vi "StorageXMutationAddTermForClose.vi"(1 "Node type":T4(ring), 2 "TermSpecs in":T1[](array[typedef])) -> (0 "TermSpecs out":T1[](array[typedef]))   [LabVIEW 2017]
uses:
  <vilib>/Platform/storage/lvStorage.llb/TerminalDef.ctl
  <vilib>/Platform/storage/lvStorage.llb/_TerminalStyle.ctl
  <vilib>/Utility/XNodeSupport.llb/XRect32.ctl
  <vilib>/Platform/storage/lvStorage.llb/_dataTypeEnumForTerminals.ctl
panel:
  in  "Name":string="file path"
  in  "terminalDef":T1={"direction"=enum."Input", "typeDescriptor"="", "color"=0, "oldTerm"=0, "style"=enum."Express", "optional"=FALSE, "bounds"={"t"=0, "l"=0, "b"=138, "r"=96}, "termRefs"=[], "Name"="", "Data"=variant, "wiredTypeDescriptor"=""}
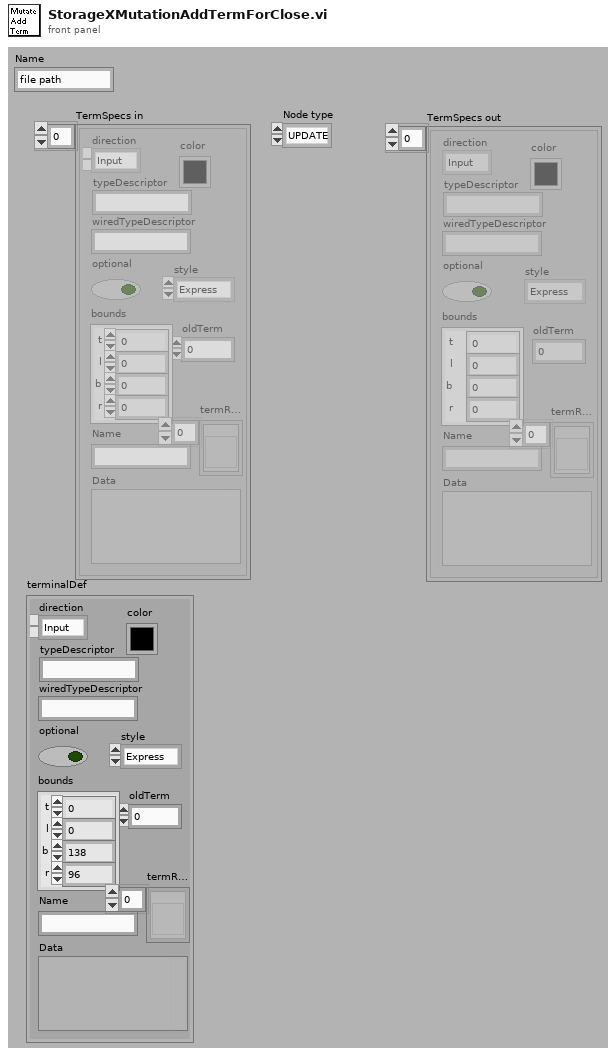
[diagram p1: front panel]
types:
  T1 = typedef "TerminalDef.ctl" = cluster{"direction":enum16{"Input", "Output"}, "typeDescriptor":string, "color":u32, "oldTerm":i32, "style":T2, "optional":bool, "bounds":T3, "termRefs":refnum<vi>[], "Name":string, "Data":variant, "wiredTypeDescriptor":string}
  T2 = typedef "_TerminalStyle.ctl" = enum16{"Express", "Collapsed", "Internal"}
  T3 = typedef "XRect32.ctl" = cluster{"t":i32, "l":i32, "b":i32, "r":i32}
  T4 = enum16{"UPDATE", "READ", "QUERY", "CREATE CHILD", "CREATE", "CONNECT", "DISCONNECT"}
  T5 = typedef "_dataTypeEnumForTerminals.ctl" = enum16{"Data Storage", "Data Object", "Root", "Channel", "Error in", "Error out", "Storage Location (path)", "Storage Location (string)", "Storage Format", "Overwrite options (enum)", "Append / Replace (enum)", "index", "count", "Comparison (enum)", "Signal", "Channelgroup", "Cluster", "DBL", "SGL", "I32", "I16", "U8", "TIME", "STRING", "ENUM", "waveform", "DDT", "DAQmx Channel"}
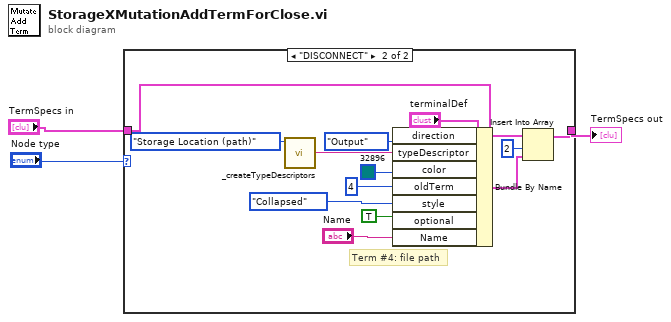
[diagram p0: block diagram]
diagram:
  n1 = case shown="\"DISCONNECT\"" "Node type" {
    tunnel: "TermSpecs in" -> [w4 w8]
    tunnel: [w4 w5] -> w2
    frame Default {
    }
    frame "DISCONNECT" {
      # "Term #4: file path"
      n2 = call <vilib>:"_createTypeDescriptors.vi"("DNL_Data type"=_dataTypeEnumForTerminals."Storage Location (path)" ("Data type")) -> ("DNL_Type descriptor"=w13:string)  [unwired: 7 in, 3 out]
      n3 = Bundle By Name(cluster="terminalDef", "direction"=enum16{"Input", "Output"}."Output", "typeDescriptor"=w13, "color"=u32 32896 ("color(black)"), "oldTerm"=4, "style"=enum16{"Express", "Collapsed"}."Collapsed", "optional"=TRUE, "Name"="Name") -> (w7:T1)
      n4 = Insert Into Array(array=w8, index=2, new element=w7) -> (w5:T1[])
    }
  }
  "TermSpecs out" <- w2
